vi "DataReader.vi"(11 "Filename":path=path "D:/Sonify Labview/Data/PorkSkin_40C_5Min.lvm") -> ()   [LabVIEW 2016]
panel:
  out "Acoustic Pressure":dbl[](graph) caption="Signals"
  out "Thermal Dose (Min)":dbl format="%#_2g"
  out "Drive Voltage":dynamicdata(graph) caption="Signals"
  out "Temperature":dynamicdata(graph) caption="Signals"
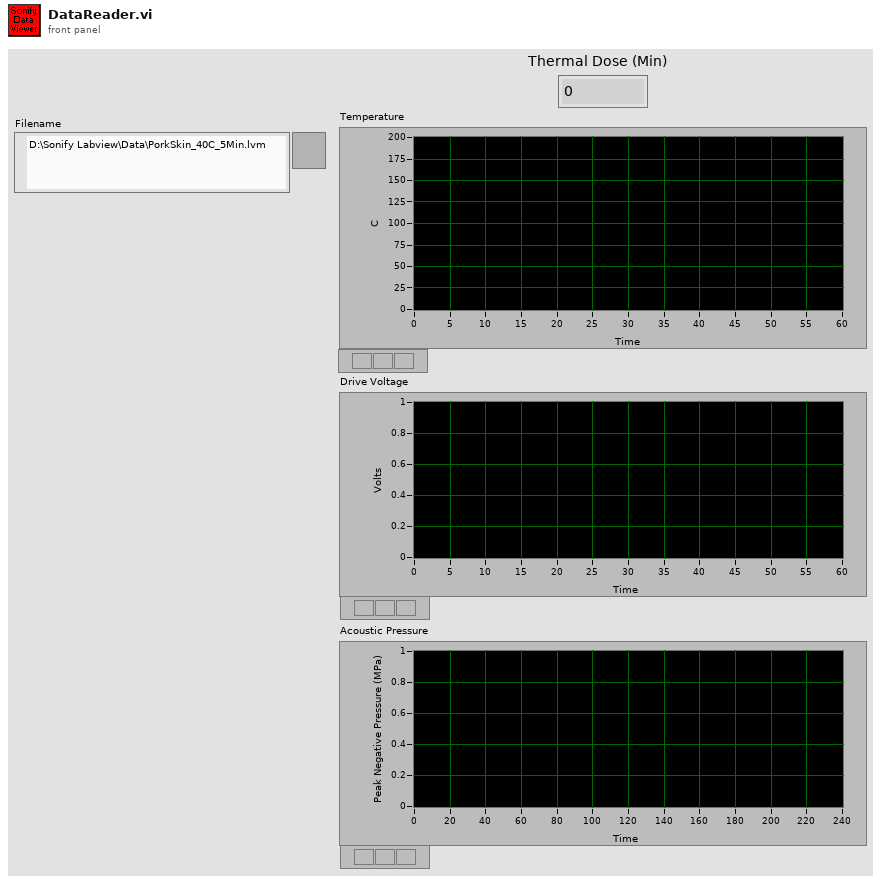
[diagram p1: front panel]
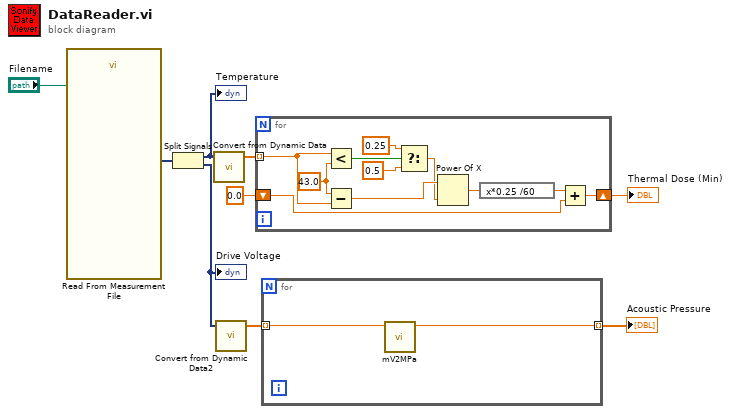
[diagram p0: block diagram]
diagram:
  n1 = call "Read From Measurement File"("Filename"="Filename") -> ("Signals"=w9:dynamicdata)  [unwired: 5 in, 5 out]
  n2 = Split Signals(w9) -> (w7:dynamicdata, w3:dynamicdata)  [unwired: 2 in]
  "Temperature" <- w7
  "Drive Voltage" <- w3
  n3 = call "Convert from Dynamic Data"("Dynamic Data Type"=w7) -> ("Array"=w6:dbl[])  [unwired: 3 in]
  n4 = call "Convert from Dynamic Data2"("Dynamic Data Type"=w3) -> ("Array"=w1:dbl[])  [unwired: 3 in]
  n5 = for {
    tunnel: w6 -> [w17] mode=indexing
    shift-right: [w14] -> w4
    shift-left: 0.0 -> [w13]
    w10 = 43.0 ("y")
    n6 = Less?(x=w17, y=w10) -> (x < y?=w20:bool)
    n7 = Subtract(x=w10, y=w17) -> (x-y=w12:dbl)
    n8 = Select(t=0.25, s=w20, f=0.5) -> (s? t:f=w11:dbl)
    n9 = Power Of X(1:w11, 2:w12) -> (0:w16:dbl)
    n10 = expression code="x*0.25 /60"(w16) -> (w15:dbl)
    n11 = Add(x=w15, y=w13) -> (x+y=w14:dbl)
  }
  "Thermal Dose (Min)" <- w4
  n12 = for {
    tunnel: [w21] -> w2 mode=indexing
    tunnel: w1 -> [w22] mode=indexing
    n13 = call "mV2MPa.vi"("Volts In"=w22) -> ("MPa Out"=w21:dbl)  [unwired: 10 in]
  }
  "Acoustic Pressure" <- w2
